vi "未命名 2.vi"() -> ()   [LabVIEW 2013]
panel:
  out "连接的字符串":string
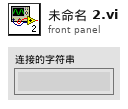
[diagram p1: front panel]
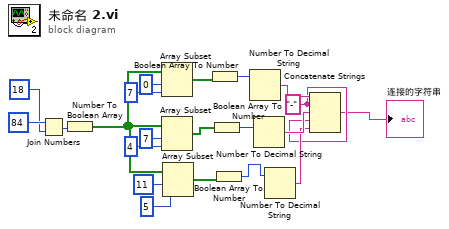
[diagram p0: block diagram]
diagram:
  w10 = "-" ("字符串")
  n1 = Join Numbers(hi=u8 84, lo=u8 18 ("hi")) -> ((hi.lo)=w21:u16)
  n2 = Number To Boolean Array(number=w21) -> (Boolean array=w20:bool[])
  n3 = Array Subset(array=w20, index=0 ("索引"), length=7 ("长度")) -> (w19:bool[])
  n4 = Array Subset(array=w20, index=7 ("索引"), length=4 ("长度")) -> (w18:bool[])
  n5 = Array Subset(array=w20, index=11 ("索引"), length=5 ("长度")) -> (w17:bool[])
  n6 = Boolean Array To Number(Boolean array=w19) -> (number=w16:u32)
  n7 = Boolean Array To Number(Boolean array=w18) -> (number=w14:u32)
  n8 = Boolean Array To Number(Boolean array=w17) -> (number=w13:u32)
  n9 = Number To Decimal String(number=w16) -> (decimal integer string=w15:string)  [unwired: 1 in]
  n10 = Number To Decimal String(number=w14) -> (decimal integer string=w12:string)  [unwired: 1 in]
  n11 = Number To Decimal String(number=w13) -> (decimal integer string=w11:string)  [unwired: 1 in]
  n12 = Concatenate Strings(w15, w10, w12, w10, w11) -> (→"连接的字符串":string)
